vi "UART Open.vi"(8 "Error In":errorcluster, 9 "Baud Rate (9600)":u32=9600, 10 "UART Channel (0)":u8, 11 "LINX Resource":T1) -> (0 "Error Out":errorcluster, 3 "LINX Resource":T1)   [LabVIEW 2011, in "LVH-LINX.lvlib"]
doc: "Open the UART channel with the specified baud rate."
uses:
  LVH-LINX.lvlib
  Private/Type Defs/LINX Ref.ctl
  Private/Type Defs/Platform.ctl
  Private/Type Defs/Interface.ctl
  Private/Device/Type Defs/LINX Device Config.ctl
  Private/Device/Type Defs/TCP Config.ctl
  Private/Device/Type Defs/Channels.ctl
  Private/Type Defs/Peripheral.ctl
  Private/Type Defs/Channel FGV States.ctl
  <vilib>/Instr/_visa.llb/VISA Configure Serial Port (Instr).vi
  Private/Device/Device.lvlib
  Private/myRIO/myRIO.lvlib
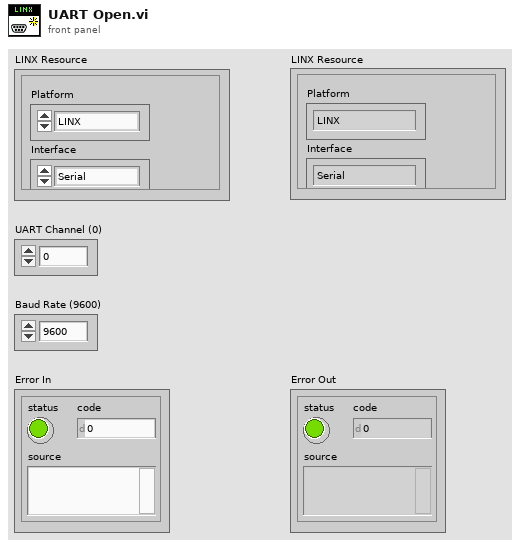
[diagram p1: front panel]
types:
  T1 = typedef "LVH-LINX.lvlib/LINX Ref.ctl" = cluster{"Platform":T2, "Interface":T3, "LINX Device Config":T4}
  T2 = typedef "LVH-LINX.lvlib/Platform.ctl" = enum16{"LINX", "myRIO"}
  T3 = typedef "LVH-LINX.lvlib/Interface.ctl" = enum16{"Serial", "TCP"}
  T4 = typedef "LVH-LINX.lvlib/Device.lvlib/LINX Device Config.ctl" = cluster{"Interface":T3, "COM Port":refnum<visa-resource-name>, "TCP Configuration":T5, "Device Family":u8, "Device ID":u8, "Device Name":string, "TCP Ref":refnum<k5>, "Channels":T6}
  T5 = typedef "LVH-LINX.lvlib/Device.lvlib/TCP Config.ctl" = cluster{"IP Address":string, "Port":u16}
  T6 = typedef "LVH-LINX.lvlib/Channels.ctl" = cluster{"DI":u8[], "DO":u8[], "AI":u8[], "AO":u8[], "PWM":u8[], "QE":u8[], "UART":u8[], "I2C 2":u8[], "SPI":u8[], "CAN":u8[], "Servo":u8[], "AI Ref (V)":dbl, "AO Ref (V)":dbl, "AO Resolution (Bits)":u8}
  T7 = typedef "LVH-LINX.lvlib/Peripheral.ctl" = enum8{"DI", "DO", "AI", "AO", "PWM", "QE", "UART", "I2C", "SPI", "CAN", "Servo"}
  T8 = typedef "LVH-LINX.lvlib/Channel FGV States.ctl" = enum16{"Initialize", "Get", "Set"}
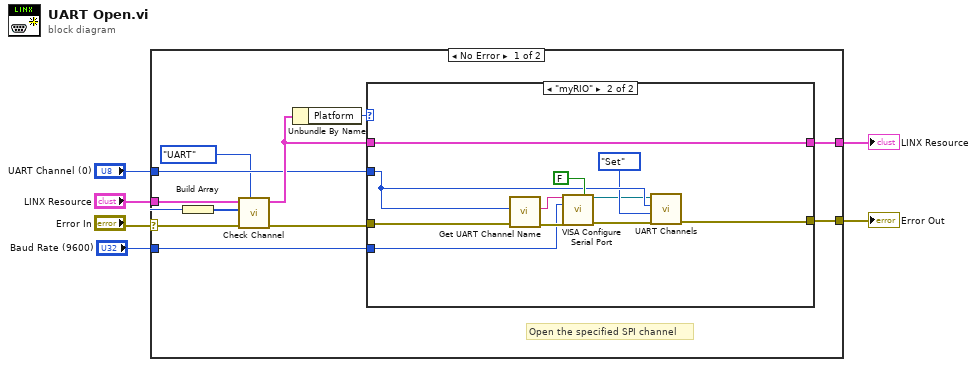
[diagram p0: block diagram]
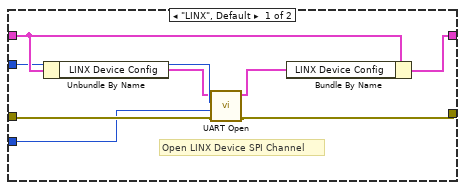
[diagram p2: hidden frame]
diagram:
  n1 = case shown="No Error" "Error In" {
    selector: "Error In" -> [w7 w38]
    tunnel: [w16 w38] -> w6
    tunnel: [w15 w37] -> w5
    tunnel: "LINX Resource" -> [w14 w37]
    tunnel: "UART Channel (0)" -> [w10 _]
    tunnel: "Baud Rate (9600)" -> [w8 _]
    frame No Error {
      # "Open the specified SPI channel"
      n2 = Build Array(w10) -> (w11:u8[])
      n3 = call "Check Channel.vi"("Peripheral"=Peripheral."UART", "Error In"=w7, "Channels"=w11, "LINX Resource"=w14) -> ("Error Out"=w12:errorcluster, "LINX Resource"=w13:T1)  [unwired: 5 in, 1 out]
      n4 = Unbundle By Name(w13) -> ("Platform"=w17:T2)
      n5 = case shown="\"myRIO\"" w17 {
        tunnel: w12 -> [w22 w29]
        tunnel: w13 -> [w25 w36]
        tunnel: [w23 w27] -> w16
        tunnel: [w24 w36] -> w15
        tunnel: w10 -> [w21 w31]
        tunnel: w8 -> [w20 w33]
        frame "LINX", Default {
          # "Open LINX Device SPI Channel"
          n6 = Unbundle By Name(w25) -> ("LINX Device Config"=w19:T4)
          n7 = call "UART Open.vi"("Error In"=w22, "Baud Rate (9600)"=w20, "UART Channel"=w21, "LINX Device Config"=w19) -> ("Error Out"=w23:errorcluster, "LINX Device Config"=w18:T4)  [unwired: 6 in]
          n8 = Bundle By Name(cluster=w25, "LINX Device Config"=w18) -> (w24:T1)
        }
        frame "myRIO" {
          n9 = call "Get UART Channel Name.vi"("Error In"=w29, "UART Channel"=w31) -> ("Error Out"=w34:errorcluster, "UART Channel"=w32:string)  [unwired: 8 in]
          n10 = call-poly "VISA Configure Serial Port"("VISA resource name"=w32, "Enable Termination\nChar (T)"=FALSE ("Enable Termination\nChar (T)"), "baud rate (9600)"=w33, "error in (no error)"=w34) -> ("VISA resource name out"=w26:refnum<visa-resource-name>, "error out"=w28:errorcluster)  [unwired: 10 in]
          n11 = call "UART Channels.vi"("Error In"=w28, "Channel State"=Channel_FGV_States."Set", "Channel Number"=w31, "UART Channel"=w26) -> ("Error Out"=w27:errorcluster)  [unwired: 6 in, 1 out]
        }
      }
    }
    frame Error {
    }
  }
  "Error Out" <- w6
  "LINX Resource" <- w5
